vi "onTestExecution.vi"(6 "timeout (2000 ms)":i32=2000, 7 "Name":string, 8 "error in (no error)":errorcluster, 11 "Test Runner.Template in":refnum<class "caraya unit tests.lvclass">) -> (0 "error out":errorcluster, 3 "Test Runner.Template out":refnum<class "caraya unit tests.lvclass">)   [LabVIEW 2023, in "caraya unit tests.lvclass"]
uses:
  caraya unit tests.lvclass
  caraya unit tests.lvclass/caraya unit tests.ctl
  <vilib>/addons/_JKI Toolkits/Caraya/classes/Test/Test.lvclass
  <vilib>/addons/_JKI Toolkits/Caraya/classes/Assert/Assert.lvclass
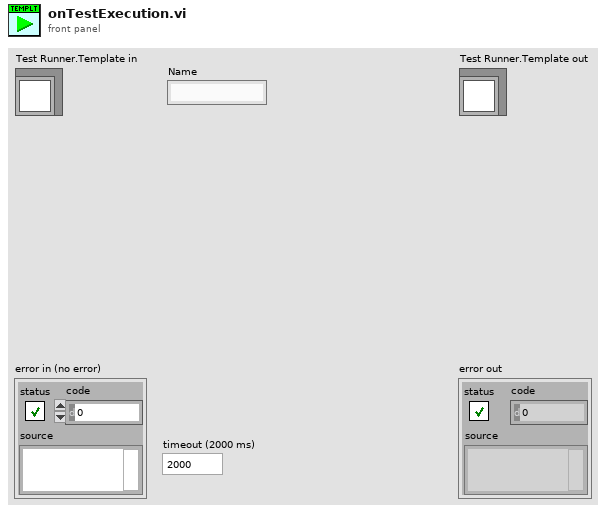
[diagram p1: front panel]
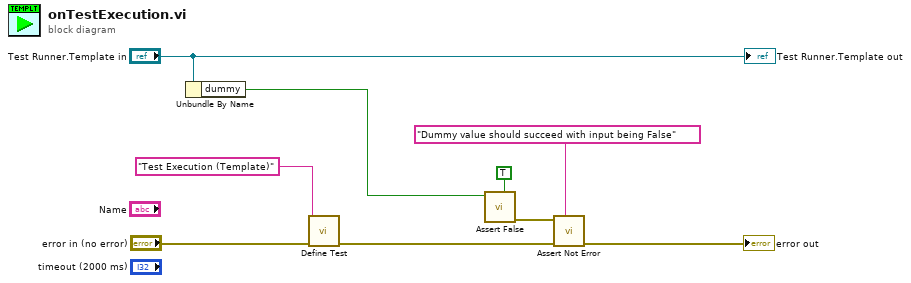
[diagram p0: block diagram]
diagram:
  n1 = Unbundle By Name("Test Runner.Template in") -> ("dummy"=w4:bool)
  n2 = call <vilib>:"Define Test.vi"("error in (no error)"="error in (no error)", "Label (VI Title)"="Test Execution (Template)") -> ("error out"=w3:errorcluster)  [unwired: 8 in, 1 out]
  n3 = call <vilib>:"Assert False.vi"("Assert Only? (F)"=TRUE, "False?"=w4) -> ("error out"=w7:errorcluster)  [unwired: 8 in, 1 out]
  n4 = call <vilib>:"Assert Not Error.vi"("Label"="Dummy value should succeed with input being False", "error in (no error)"=w3, "Not Error?"=w7) -> ("error out"=→"error out":errorcluster)  [unwired: 7 in, 1 out]
  "Test Runner.Template out" <- "Test Runner.Template in"
